vi "Teleop.vi"(10 "Match Info":T1={"Autonomous Elapsed Seconds"=0.0, "TeleOp Elapsed Seconds"=0.0, "Disabled Elapsed Seconds"=0.0, "Visited Autonomous"=FALSE, "Visited TeleOp"=FALSE, "Visited Disabled"=FALSE, "Autonomous Settings"={"Autonomous Style"=enum."Independent", "VI Refnum"=refnum}}, 11 "Call Context":T2) -> ()   [LabVIEW 2016]
doc: "This VI is called for each TeleOp packet received from the DS where the robot is not disabled. It is often used to read from the joysticks and update I/O or to update setpoints for timed control loops. It should complete and return within 20 milliseconds or it may miss DS packets."
uses:
  <vilib>/Rock Robotics/WPI/DriverStation/WPI_DriverStationDerivedRobotMode.ctl
  <vilib>/Rock Robotics/WPI/DriverStation/WPI_DriverStationMatch Info.ctl
  TypeDef/ENUM_Joystick_Buttons.ctl
  TypeDef/ENUM_Joystick_Axes.ctl
  TypeDef/CLUSTER_CMD_WC_Drive.ctl
  TypeDef/ENUM_WC_Drive_DriveMode.ctl
  TypeDef/CLUSTER_Drive_ACT Loop_VBus Data.ctl
  TypeDef/CLUSTER_X and Y.ctl
  TypeDef/CLUSTER_Drive_ACT Loop_Profile Data.ctl
  Systems/joystick/Global_Joystick Write_Data.vi
  Globals/Global_CMD_Gear.vi
  Globals/Global_CMD_Drive.vi
  Systems/Gear Pickup/CMD_GearPickup.vi
  Systems/joystick/Joystick.lvlib
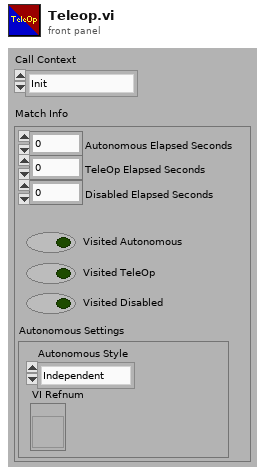
[diagram p1: front panel]
types:
  T1 = typedef "WPI_DriverStationMatch Info.ctl" = cluster{"Autonomous Elapsed Seconds":dbl, "TeleOp Elapsed Seconds":dbl, "Disabled Elapsed Seconds":dbl, "Visited Autonomous":bool, "Visited TeleOp":bool, "Visited Disabled":bool, "Autonomous Settings":cluster{"Autonomous Style":enum16{"Iterative", "Independent"}, "VI Refnum":refnum<vi>}}
  T2 = typedef "WPI_DriverStationDerivedRobotMode.ctl" = enum16{"Init", "Execute", "Stop"}
  T3 = typedef "ENUM_Joystick_Buttons.ctl" = enum16{"Green A", "Red B", "Blue X", "Yellow Y", "Left Bumper", "Right Bumper", "Back", "Start", "Left Joystick", "Right Joystick"}
  T4 = typedef "CLUSTER_CMD_WC_Drive.ctl" = cluster{"Drive_Mode":T5, "VBus":T6, "Profile":T8}
  T5 = typedef "ENUM_WC_Drive_DriveMode.ctl" = enum16{"Motion Profile", "VBus", "Stop"}
  T6 = typedef "CLUSTER_Drive_ACT Loop_VBus Data.ctl" = cluster{"Drive":T7, "Turbo":bool}
  T7 = typedef "CLUSTER_X and Y.ctl" = cluster{"Steer":dbl, "Throtle":dbl}
  T8 = typedef "CLUSTER_Drive_ACT Loop_Profile Data.ctl" = cluster{"Start":bool}
  T9 = typedef "ENUM_Joystick_Axes.ctl" = enum16{"Left X", "Left Y", "Left Trigger", "Right Trigger", "Right X", "Right Y"}
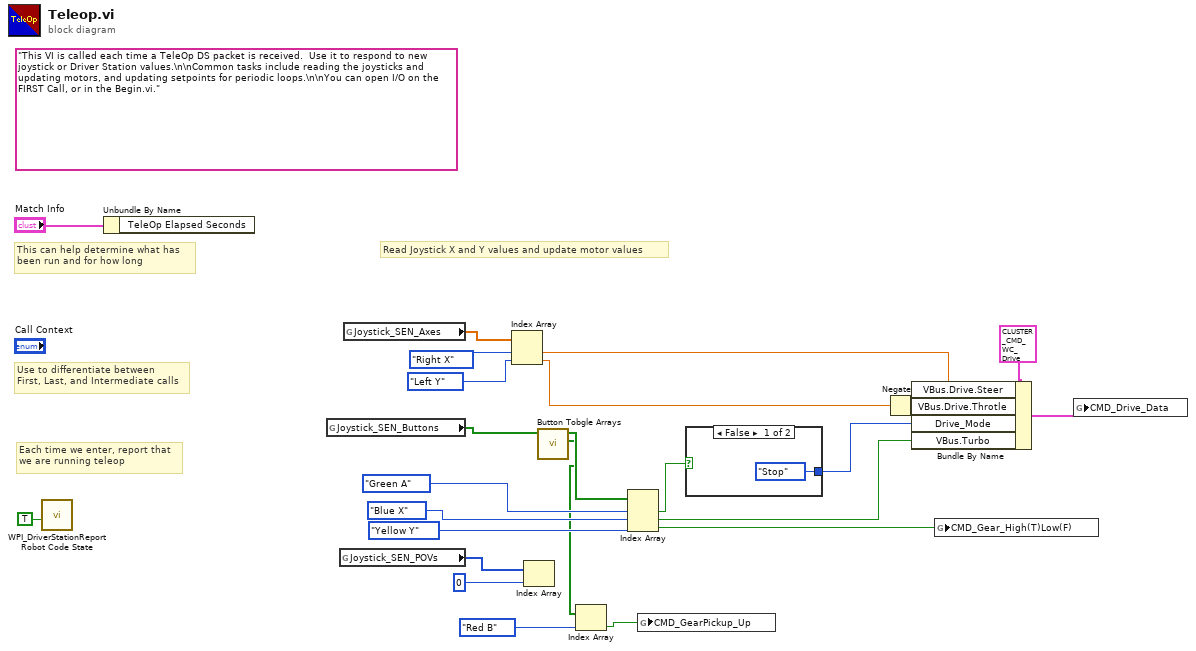
[diagram p0: block diagram]
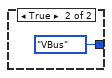
[diagram p2: hidden frame]
diagram:
  (unwired) "This VI is called each time a TeleOp DS packet is received.  Use it to respond to new joystick or Driver Station values.\n\nCommon tasks include reading the joysticks and updating motors, and updating setpoints for periodic loops.\n\nYou can open I/O on the FIRST Call, or in the Begin.vi."
  # "Each time we enter, report that\nwe are running teleop"
  # "Use to differentiate between\nFirst, Last, and Intermediate calls"
  # "This can help determine what has\nbeen run and for how long"
  # "Read Joystick X and Y values and update motor values"
  n1 = call <vilib>:"WPI_DriverStationReport Robot Code State.vi"("TeleOp"=TRUE ("Autonomous")) -> ()  [unwired: 10 in, 1 out]
  n2 = Unbundle By Name("Match Info") -> ()  [unwired: 1 out]
  n3 = global read "Global_Joystick Write_Data.vi" "Joystick_SEN_Buttons"() -> (w11:bool[])
  n4 = global read "Global_Joystick Write_Data.vi" "Joystick_SEN_POVs"() -> (w21:i16[])
  n5 = global read "Global_Joystick Write_Data.vi" "Joystick_SEN_Axes"() -> (w22:dbl[])
  n6 = Index Array(array=w22, index #1=ENUM_Joystick_Axes."Right X" ("Joystick_Axes"), index #2=ENUM_Joystick_Axes."Left Y" ("Joystick_Axes")) -> (element #1=w6:dbl, element #2=w4:dbl)
  n7 = Index Array(array=w21, index=0) -> ()  [unwired: 1 out]
  n8 = call "Button Tobgle Arrays.vi"("Joystick_SEN_Buttons"=w11) -> ("Rizing Edge Outputs Out"=w3:bool[], "Toggle Outputs Out"=w14:bool[])  [unwired: 8 in, 1 out]
  n9 = Index Array(array=w3, index=ENUM_Joystick_Buttons."Red B" ("Joystick_Buttons")) -> (element=w1:bool)
  n10 = Index Array(array=w14, index #1=ENUM_Joystick_Buttons."Green A" ("Joystick_Buttons"), index #2=ENUM_Joystick_Buttons."Blue X" ("Joystick_Buttons"), index #3=ENUM_Joystick_Buttons."Yellow Y" ("Joystick_Buttons")) -> (element #1=w13:bool, element #2=w9:bool, element #3=w7:bool)
  n11 = global write "CMD_GearPickup.vi" "CMD_GearPickup_Up"(w1) -> ()
  n12 = case shown="False" w13 {
    tunnel: [ENUM_WC_Drive_DriveMode."Stop" ("CMD_Drive_Mode") ENUM_WC_Drive_DriveMode."VBus" ("CMD_Drive_Mode")] -> w12
    frame False {
    }
    frame True {
    }
  }
  n13 = Negate(x=w4) -> (-x=w5:dbl)
  n14 = Bundle By Name(cluster=T4 {"Drive_Mode"=enum."Motion Profile", "VBus"={"Drive"={"Steer"=0.0, "Throtle"=0.0}, "Turbo"=FALSE}, "Profile"={"Start"=FALSE}} ("CMD_DriveCluster"), "VBus.Drive.Steer"=w6, "VBus.Drive.Throtle"=w5, "Drive_Mode"=w12, "VBus.Turbo"=w9) -> (w17:T4)
  n15 = global write "Global_CMD_Gear.vi" "CMD_Gear_High(T)Low(F)"(w7) -> ()
  n16 = global write "Global_CMD_Drive.vi" "CMD_Drive_Data"(w17) -> ()
